vi "tbcontrol1.vi"() -> ()   [LabVIEW 2021]
panel:
  in  "Page Visible":bool
  in  "stop":bool
  in  "Tab Control":enum32{"Page 1", "Page 2"}(tab)
  out "x*y":dbl
  out "Waveform Chart":dbl(graph)
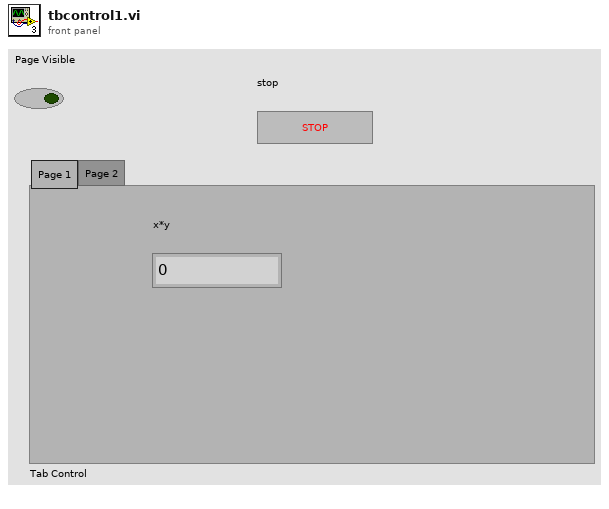
[diagram p1: front panel]
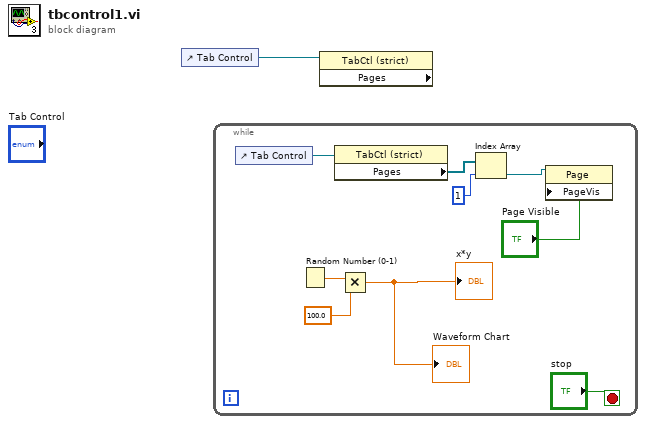
[diagram p0: block diagram]
diagram:
  n1 = control-ref of="Tab Control"() -> (w1:refnum<vi>)
  n2 = while {
    stop <- "stop" stop-if-true
    n3 = control-ref of="Tab Control"() -> (w6:refnum<vi>)
    n4 = Random Number (0-1)() -> (number: 0 to 1=w10:dbl)
    n5 = property class="TabCtl (strict)"(reference=w6) -> ("Pages"=w5:refnum<vi>[])  [unwired: 1 in, 2 out]
    n6 = Multiply(x=w10, y=100.0) -> (x*y=→"x*y" →"Waveform Chart":dbl)
    n7 = Index Array(array=w5, index=1) -> (element=w4:refnum<vi>)
    n8 = property class="Page"(reference=w4, "PageVis"="Page Visible") -> ()  [unwired: 1 in, 2 out]
  }
  n9 = property class="TabCtl (strict)" props=["Pages"](reference=w1) -> ()  [unwired: 1 in, 3 out]
